vi "Sub_Pin_Location_to_Node.vi"(10 "Pin Location":dbl, 11 "Experiment in":T1) -> (3 "DOF of Interest":i32)   [LabVIEW 2021]
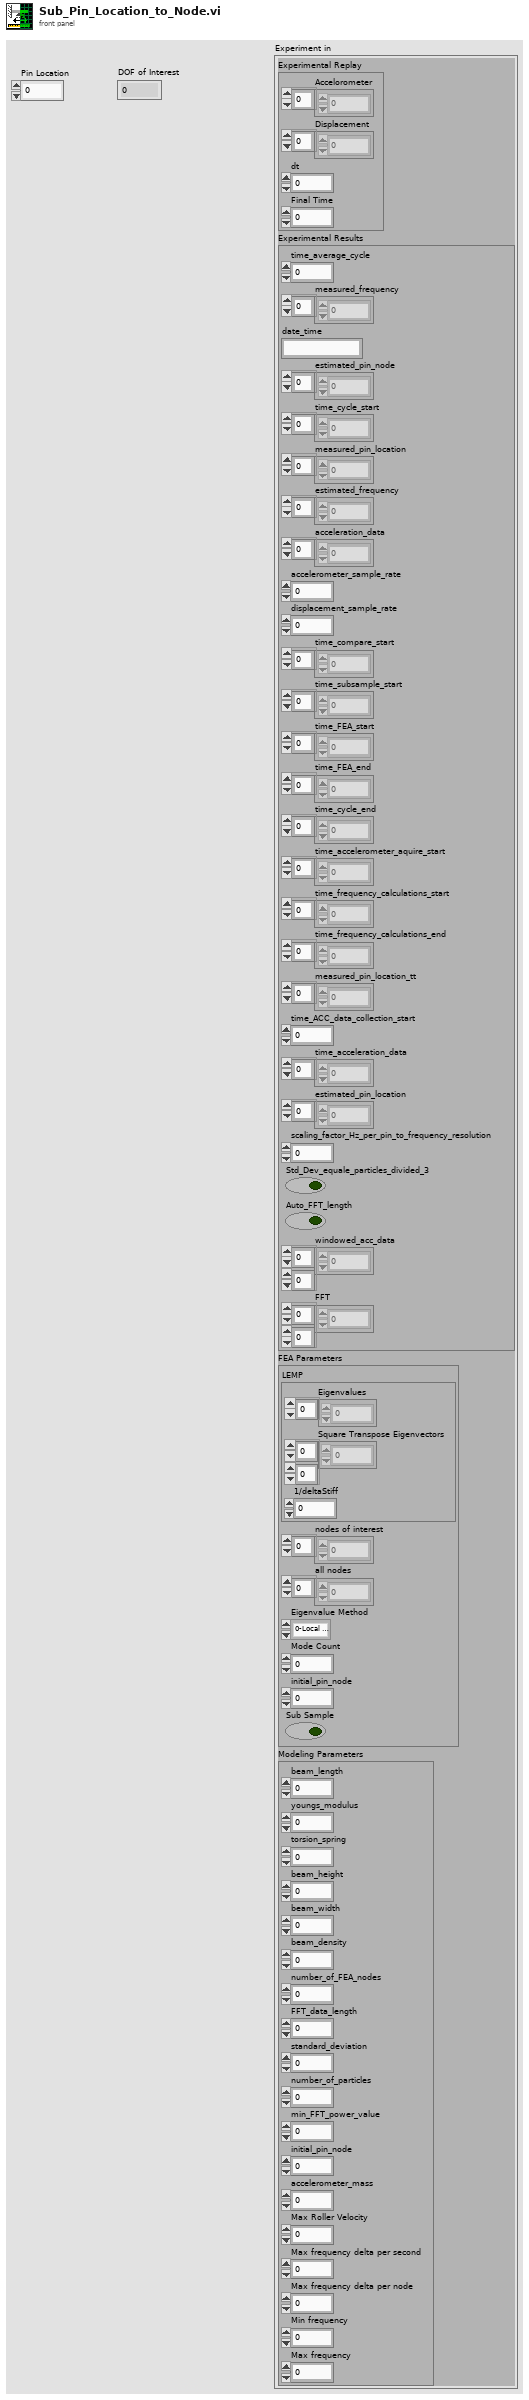
[diagram p1: front panel]
types:
  T1 = cluster{"Experimental Replay":cluster{"Accelorometer":dbl[], "Displacement":dbl[], "dt":dbl, "Final Time":dbl}, "Experimental Results":cluster{"time_average_cycle":dbl, "measured_frequency":dbl[], "date_time":string, "estimated_pin_node":i32[], "time_cycle_start":dbl[], "measured_pin_location":dbl[], "estimated_frequency":dbl[], "acceleration_data":dbl[], "accelerometer_sample_rate":dbl, "displacement_sample_rate":dbl, "time_compare_start":dbl[], "time_subsample_start":dbl[], "time_FEA_start":dbl[], "time_FEA_end":dbl[], "time_cycle_end":dbl[], "time_accelerometer_aquire_start":dbl[], "time_frequency_calculations_start":dbl[], "time_frequency_calculations_end":dbl[], "measured_pin_location_tt":dbl[], "time_ACC_data_collection_start":dbl, "time_acceleration_data":dbl[], "estimated_pin_location":dbl[], "scaling_factor_Hz_per_pin_to_frequency_resolution":dbl, "Std_Dev_equale_particles_divided_3":bool, "Auto_FFT_length":bool, "windowed_acc_data":dbl[][], "FFT":dbl[][]}, "FEA Parameters":cluster{"LEMP":cluster{"Eigenvalues":dbl[], "Square Transpose Eigenvectors":dbl[][], "1/deltaStiff":dbl}, "nodes of interest":i32[], "all nodes":i32[], "Eigenvalue Method":enum16{"0-Local Eigen Modification Procedure", "1-LabVIEW generalized eigenvalues", "2-LabVIEW M^-1K eigenvalues", "3-LabVIEW Cholesky Factorization", "4-Cholesky Factorization CPU SGL", "5-Cholesky Factorization CPU FXP", "6-Cholesky Factorization FPGA SGL", "7-Cholesky Factorization FPGA SGL SCL"}, "Mode Count":i32, "initial_pin_node":i32, "Sub Sample":bool}, "Modeling Parameters":cluster{"beam_length":dbl, "youngs_modulus":dbl, "torsion_spring":dbl, "beam_height":dbl, "beam_width":dbl, "beam_density":dbl, "number_of_FEA_nodes":i32, "FFT_data_length":i32, "standard_deviation":dbl, "number_of_particles":i32, "min_FFT_power_value":dbl, "initial_pin_node":i32, "accelerometer_mass":dbl, "Max Roller Velocity":dbl, "Max frequency delta per second":dbl, "Max frequency delta per node":dbl, "Min frequency":dbl, "Max frequency":dbl}}
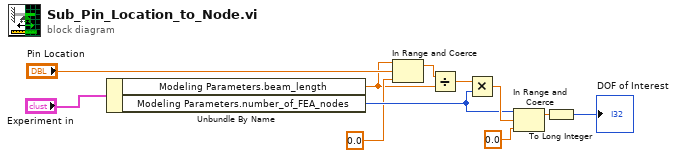
[diagram p0: block diagram]
diagram:
  n1 = Unbundle By Name("Experiment in") -> ("Modeling Parameters.beam_length"=w1:dbl, "Modeling Parameters.number_of_FEA_nodes"=w7:i32)
  n2 = In Range and Coerce(upper limit=w1, x="Pin Location", lower limit=0.0) -> (coerced(x)=w3:dbl)  [unwired: 1 out]
  n3 = Divide(x=w3, y=w1) -> (x/y=w9:dbl)
  n4 = Multiply(x=w9, y=w7) -> (x*y=w8:dbl)
  n5 = In Range and Coerce(upper limit=w7, x=w8, lower limit=0.0) -> (coerced(x)=w10:dbl)  [unwired: 1 out]
  n6 = To Long Integer(number=w10) -> (32bit integer=→"DOF of Interest":i32)
